vi "send_serial_command.vi"(8 "error in (no error)":errorcluster, 10 "Command":string="*IDN?", 11 "VISA resource name":refnum<visa-resource-name>="COM5") -> (0 "error out":errorcluster, 3 "Response":string)   [LabVIEW 2020]
uses:
  Program Files/National Instruments/LabVIEW 2020/examples/Instrument IO/Serial/support/Serial - Settings.ctl
  Program Files/National Instruments/LabVIEW 2020/examples/Instrument IO/Serial/support/Serial - XON-XOFF Characters.ctl
  Program Files/National Instruments/LabVIEW 2020/examples/Instrument IO/Serial/support/Serial - ASCII Characters.ctl
  <vilib>/Instr/_visa.llb/VISA Configure Serial Port (Instr).vi
panel:
  in  "Termination Character":u8=10 format="%.0x"
  in  "End Write on Termination Character?":bool=TRUE
  in  "XON/XOFF Characters":T1={"XON"=enum."DC1", "XOFF"=enum."DC3"}
  in  "Serial Settings":T3={"baud rate"=9600, "data bits"=8, "parity"=enum."None", "stop bits"=10, "flow control"=0} {"flow control" items=["None"=0, "XON/XOFF"=1, "RTS/CTS"=2, "DTR/DSR"=4]; "stop bits" items=["1.0"=10, "1.5"=15, "2.0"=20]; "data bits" min=5 max=8 step=1; "baud rate" items=["75"=75, "110"=110, "134"=134, "150"=150, "300"=300, "600"=600, "1200"=1200, "1800"=1800, "2400"=2400, "4800"=4800, "7200"=7200, "9600"=9600, "14400"=14400, "19200"=19200, "28800"=28800, "38400"=38400, "56000"=56000, "57600"=57600, "115200"=115200, "128000"=128000, "230400"=230400]}
  in  "End Read on Termination Character?":bool=TRUE
  in  "Read Count":u32=1000
  in  "Read":bool=TRUE
  in  "Stop":bool
  in  "Write":bool=TRUE
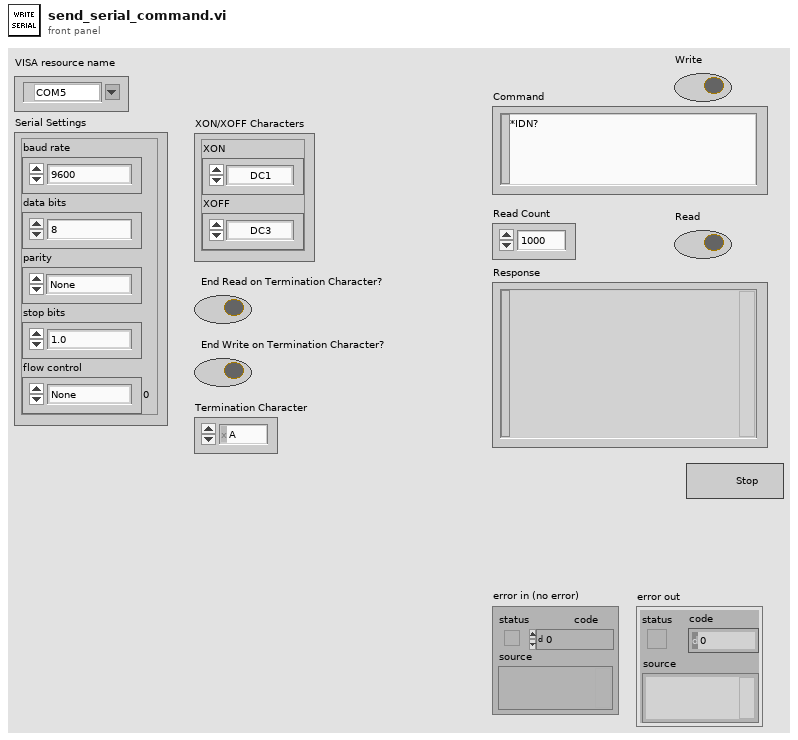
[diagram p1: front panel]
types:
  T1 = typedef "Serial - XON-XOFF Characters.ctl" = cluster{"XON":T2, "XOFF":T2}
  T2 = typedef "Serial - ASCII Characters.ctl" = enum16{"NUL", "SOH", "STX", "ETX", "EOT", "ENQ", "ACK", "BEL", "BS", "HT", "LF", "VT", "FF", "CR", "SO", "SI", "DLE", "DC1", "DC2", "DC3", "DC4", "NAK", "SYN", "ETB", "CAN", "EM", "SUB", "ESC", "FS", "GS", "RS", "US", "SP", "!", "\"", "#", "$", "%", "&", "'", "(", ")", "*", "+", ",", "- (-)", ".", "/", "0", "1", "2", "3", "4", "5", "6", "7", "8", "9", ":", ";", "<", "=", ">", "?", "@", "A", "B", "C", "D", "E", "F", "G", "H", "I", "J", "K", "L", "M", "N", "O", "P", "Q", "R", "S", "T", "U", "V", "W", "X", "Y", "Z", "[", "\\", "]", "^", "_", "`", "a", "b", "c", "d", "e", "f", "g", "h", "i", "j", "k", "l", "m", "n", "o", "p", "q", "r", "s", "t", "u", "v", "w", "x", "y", "z", "{", "|", "}", "~"}
  T3 = typedef "Serial - Settings.ctl" = cluster{"baud rate":u32, "data bits":u16, "parity":enum16{"None", "Odd", "Even", "Mark", "Space"}, "stop bits":u16, "flow control":u16}
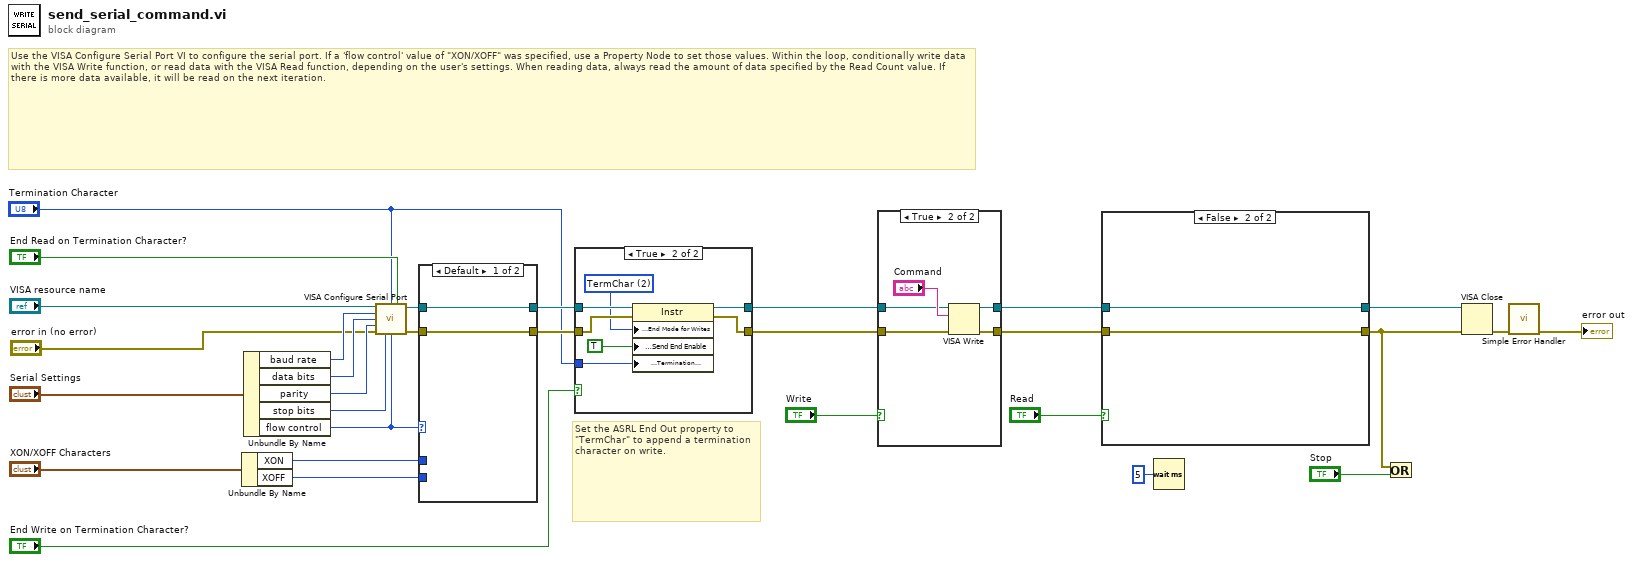
[diagram p0: block diagram]
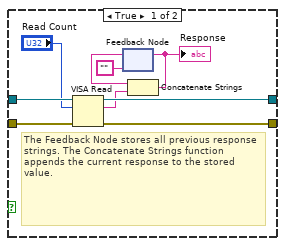
[diagram p3: hidden frame]
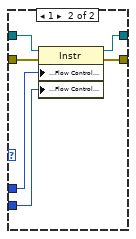
[diagram p5: hidden frame]
diagram:
  # "Set the ASRL End Out property to \"TermChar\" to append a termination character on write."
  # "Use the VISA Configure Serial Port VI to configure the serial port. If a 'flow control' value of \"XON/XOFF\" was specified, use a Property Node to set those values. Within the loop, conditionally write data with the VISA Write function, or read data with the VISA Read function, depending on the user's settings. When reading data, always read the amount of data specified by the Read Count value. If there is more data available, it will be read on the next iteration."
  n1 = Unbundle By Name("XON/XOFF Characters") -> ("XON"=w16:T2, "XOFF"=w15:T2)
  n2 = Unbundle By Name("Serial Settings") -> ("baud rate"=w23:u32, "data bits"=w24:u16, "parity"=w25:enum16{"None", "Odd", "Even", "Mark", "Space"}, "stop bits"=w26:u16, "flow control"=w17:u16)
  n3 = call-poly "VISA Configure Serial Port"("VISA resource name"="VISA resource name", "termination char\n(0xA = '\\n' = LF)"="Termination Character", "Enable Termination\nChar (T)"="End Read on Termination Character?", "baud rate (9600)"=w23, "data bits (8)"=w24, "parity (0:none)"=w25, "error in (no error)"="error in (no error)", "stop bits (10: 1 bit)"=w26, "flow control (0:none)"=w17) -> ("VISA resource name out"=w27:refnum<visa-resource-name>, "error out"=w28:errorcluster)  [unwired: 1 in, 4 out]
  n4 = case shown="Default" w17 {
    tunnel: [w31 w38] -> w14
    tunnel: [w32 w37] -> w12
    tunnel: w28 -> [w31 w36]
    tunnel: w27 -> [w32 w35]
    tunnel: w16 -> [_ w34]
    tunnel: w15 -> [_ w33]
    frame Default {
    }
    frame 1 {
      n5 = property class="Instr"(reference=w35, error in=w36, "Serial Settings:Flow Control XON Character"=w34, "Serial Settings:Flow Control XOFF Character"=w33) -> (reference out=w37:refnum<visa-resource-name>, error out=w38:errorcluster)
    }
  }
  n6 = case shown="True" "End Write on Termination Character?" {
    tunnel: w12 -> [w39 w47]
    tunnel: w14 -> [w40 w46]
    tunnel: [w39 w45] -> w11
    tunnel: [w40 w44] -> w13
    tunnel: "Termination Character" -> [_ w42]
    frame False {
    }
    frame True {
      w43 = u16 2 items=["None", "LastBit", "TermChar", "Break"] ("Serial Settings:Serial End Mode for Writes")
      n7 = property class="Instr"(reference=w47, error in=w46, "Serial Settings:End Mode for Writes"=w43, "Message Based Settings:Send End Enable"=TRUE, "Message Based Settings:Termination Character"=w42) -> (reference out=w45:refnum<visa-resource-name>, error out=w44:errorcluster)
    }
  }
  n8 = case shown="True" "Write" {
    tunnel: w11 -> [w49 w53]
    tunnel: w13 -> [w48 w52]
    tunnel: [w49 w51] -> w8
    tunnel: [w48 w50] -> w7
    frame False {
    }
    frame True {
      n9 = VISA Write(VISA resource name=w53, write buffer="Command", error in (no error)=w52) -> (VISA resource name out=w51:refnum<visa-resource-name>, error out=w50:errorcluster)  [unwired: 1 out]
    }
  }
  n10 = case shown="False" "Read" {
    tunnel: [w61 w65] -> w18
    tunnel: w8 -> [w63 w65]
    tunnel: [w59 w64] -> w19
    tunnel: w7 -> [w62 w64]
    frame True {
      # "The Feedback Node stores all previous response strings. The Concatenate Strings function appends the current response to the stored value."
      n11 = VISA Read(VISA resource name=w63, byte count="Read Count", error in (no error)=w62) -> (VISA resource name out=w61:refnum<visa-resource-name>, read buffer=w58:string, error out=w59:errorcluster)  [unwired: 1 out]
      n12 = feedback #1("") -> (w57:string)
      n13 = Concatenate Strings(w57, w58) -> (w56:string)
      "Response" <- w56
      n14 = feedback-in #1(w56) -> ()
    }
    frame False {
    }
  }
  n15 = Wait (ms)(milliseconds to wait=u32 5) -> ()  [unwired: 1 out]
  n16 = Or(x=w19, y="Stop") -> ()  [unwired: 1 out]
  n17 = VISA Close(VISA resource name=w18, error in (no error)=w19) -> (error out=w20:errorcluster)
  n18 = call <vilib>:"Simple Error Handler.vi"("error in (no error)"=w20) -> ("error out"=→"error out":errorcluster)  [unwired: 1 in, 7 out]
